vi "Remove Item by name.vi"(8 "error in (no error)":errorcluster, 10 "name":string, 11 "JSON Object in":refnum<class "JSON Object.lvclass">) -> (0 "error out":errorcluster, 2 "removed":bool, 3 "JSON Object out":refnum<class "JSON Object.lvclass">)   [LabVIEW 2011, in "JSON Object.lvclass"]
doc: "Removes a <b>JSON Value</b> in a <b>JSON Object</b> by it's name.\n\nCopyright 2012 James David Powell, Shaun Rumbell and Ton Plomp\nMore information on http://lavag.org/topic/16217-cr-json-labview"
uses:
  JSON Object.lvclass
  JSON Object.lvclass/JSON Object.ctl
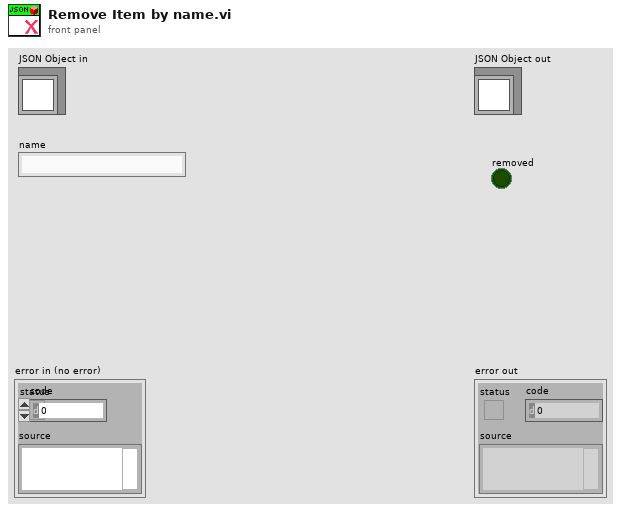
[diagram p1: front panel]
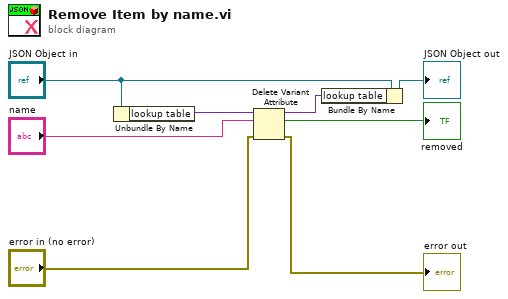
[diagram p0: block diagram]
diagram:
  n1 = Unbundle By Name("JSON Object in") -> ("lookup table"=w2:variant)
  n2 = Delete Variant Attribute(4:"error in (no error)", 6:"name", 7:w2) -> (0:→"error out":errorcluster, 2:→"removed":bool, 3:w3:variant)
  n3 = Bundle By Name(cluster="JSON Object in", "lookup table"=w3) -> (→"JSON Object out":refnum<class "JSON Object.lvclass">)
